vi "LCR_OpenShortCompensation.vi"(4 "ESR":dbl=0.001, 6 "Freq":dbl=10000.0, 7 "UseCorrection":bool, 8 "Z Open Mag":dbl=400000.0, 9 "ESL":dbl=2.3e-07, 10 "Phase Z Meas Deg":dbl=84.92384627594052, 11 "Mag Z Meas":dbl=0.014591886413483942) -> (0 "Z DUT":cdb=0.0012910863282707234+0.014534656693467846i, 2 "Phase Z DUT":dbl=84.9238462759405, 3 "Mag Z DUT":dbl=0.014591886413483942)   [LabVIEW 2020]
panel:
  in  "Z Open Phase Deg":dbl=-90.0
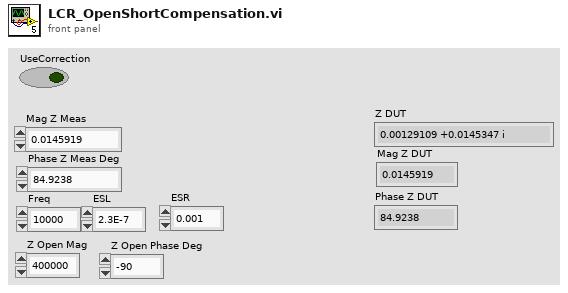
[diagram p1: front panel]
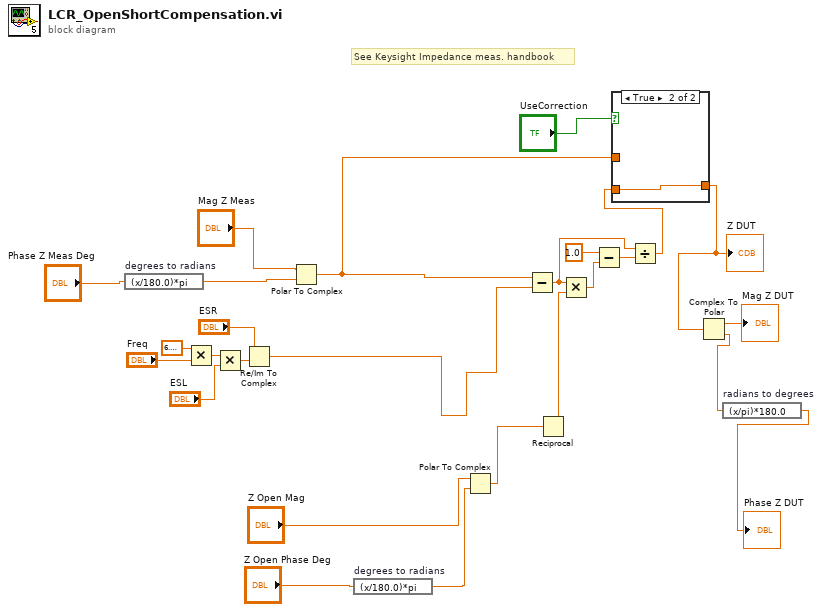
[diagram p0: block diagram]
diagram:
  # "See Keysight Impedance meas. handbook"
  n1 = expression code="(x/180.0)*pi" "degrees to radians"("Phase Z Meas Deg") -> (w14:dbl)
  n2 = Multiply(x=6.283185307179586, y="Freq") -> (x*y=w5:dbl)
  n3 = Multiply(x=w5, y="ESL") -> (x*y=w3:dbl)
  n4 = Re/Im To Complex(1:w3, 2:"ESR") -> (0:w1:cdb)
  n5 = Polar To Complex(1:w14, 2:"Mag Z Meas") -> (0:w10:cdb)
  n6 = expression code="(x/180.0)*pi" "degrees to radians"("Z Open Phase Deg") -> (w16:dbl)
  n7 = Polar To Complex(1:w16, 2:"Z Open Mag") -> (0:w18:cdb)
  n8 = Subtract(x=w10, y=w1) -> (x-y=w21:cdb)
  n9 = Reciprocal(x=w18) -> (1/x=w24:cdb)
  n10 = Multiply(x=w21, y=w24) -> (x*y=w23:cdb)
  n11 = Subtract(x=1.0, y=w23) -> (x-y=w22:cdb)
  n12 = Divide(x=w21, y=w22) -> (x/y=w12:cdb)
  n13 = case shown="True" "UseCorrection" {
    tunnel: w12 -> [_ w28]
    tunnel: [w27 w28] -> w11
    tunnel: w10 -> [w27 _]
    frame False {
    }
    frame True {
    }
  }
  "Z DUT" <- w11
  n14 = Complex To Polar(r * e^(i*theta)=w11) -> (r=→"Mag Z DUT":dbl, theta=w9:dbl)
  n15 = expression code="(x/pi)*180.0" "radians to degrees"(w9) -> (→"Phase Z DUT":dbl)
